vi "RankControls.vi"(6 "error in":errorcluster, 9 "VI Interpreter in":refnum<class "VI Interpreter.lvclass">) -> (0 "error out":errorcluster, 3 "VI Interpreter out":refnum<class "VI Interpreter.lvclass">, 4 "Rank":cluster{"nodes":i32[]}[](array[cluster]))   [LabVIEW 2014, in "Raspberry Pi Compatible Compiler for LabVIEW.lvlib" / "VI Interpreter.lvclass"]
uses:
  VI Interpreter.lvclass
  VI Interpreter.lvclass/VI Interpreter.ctl
  <vilib>/Utility/traverseref.llb/TRef TravTarget.ctl
  VI_AST/VI_AST.lvclass
  VI_AST/VI_AST.lvclass/VI_AST.ctl
  <vilib>/Utility/traverseref.llb/VI Scripting - Traverse.lvlib
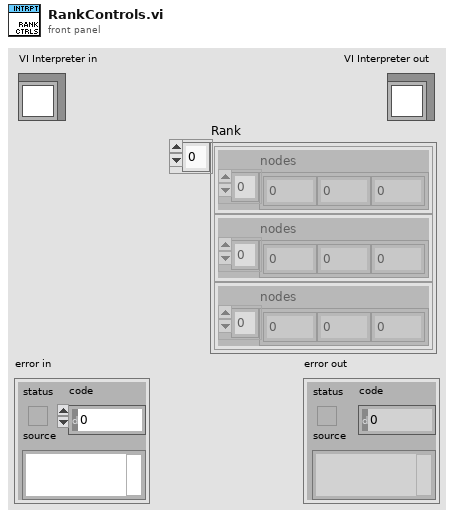
[diagram p1: front panel]
types:
  T1 = typedef "TRef TravTarget.ctl" = enum16{"FP", "BD", "Other"}
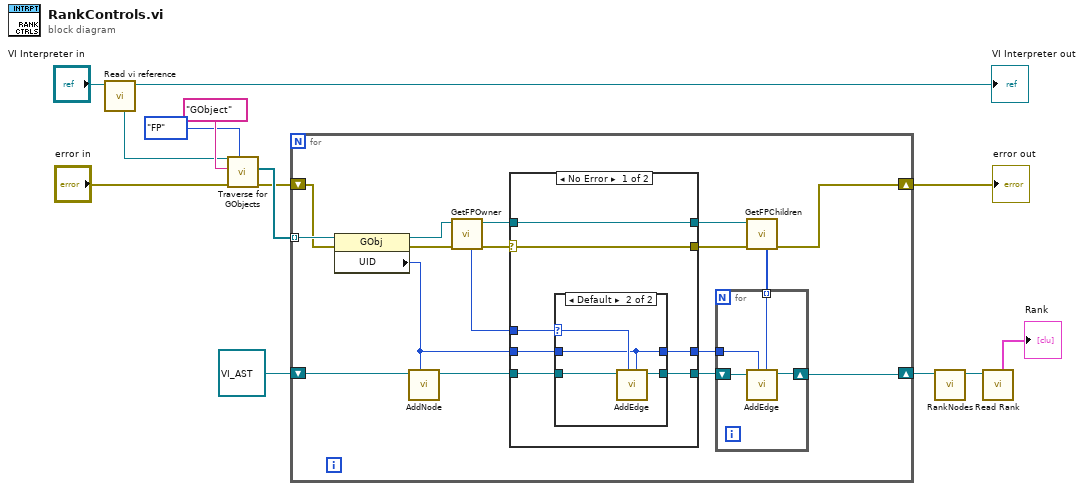
[diagram p0: block diagram]
diagram:
  n1 = call "Read vi reference.vi"("VI Interpreter in"="VI Interpreter in") -> ("VI Interpreter out"=→"VI Interpreter out":refnum<class "VI Interpreter.lvclass">, "vi reference"=w9:refnum<vi>)  [unwired: 7 in]
  n2 = call <vilib>:"Traverse for GObjects.vi"("Traverse Target"=TRef_TravTarget."FP", "error in (no error)"="error in", "Class Name"="GObject", "VI Refnum"=w9) -> ("error out"=w3:errorcluster, "References"=w4:refnum<vi>[])  [unwired: 4 in, 2 out]
  n3 = for {
    tunnel: w4 -> [w23] mode=indexing
    shift-right: [w14] -> w7
    shift-left: refnum<class "VI_AST.lvclass"> refnum ("VI_AST in") -> [w30]
    shift-right: [w18] -> w5
    shift-left: w3 -> [w22]
    n4 = property class="GObj"(reference=w23, error in=w22) -> (reference out=w26:refnum<vi>, error out=w27:errorcluster, "UID"=w28:i32)
    n5 = call "AddNode.vi"("UID"=w28, "VI_AST in"=w30) -> ("VI_AST out"=w29:refnum<class "VI_AST.lvclass">)  [unwired: 6 in, 1 out]
    n6 = call "GetFPOwner.vi"("error in"=w27, "GObj Refnum"=w26) -> ("error out"=w25:errorcluster, "GObj Refnum out"=w20:refnum<vi>, "owner UID"=w24:i32)  [unwired: 5 in]
    n7 = case shown="No Error" w25 {
      selector: w25 -> [w38 _]
      tunnel: [w41 w50] -> w17
      tunnel: w29 -> [w40 w50]
      tunnel: w28 -> [w39 w48]
      tunnel: w24 -> [w37 _]
      tunnel: [w38 _] -> w21
      tunnel: w20 -> [w36 w49]
      tunnel: [w36 w49] -> w19
      tunnel: [w35 w48] -> w15
      frame No Error {
        n8 = case shown="Default" w37 {
          selector: w37 -> [_ w45]
          tunnel: [w43 w47] -> w41
          tunnel: w40 -> [w43 w46]
          tunnel: w39 -> [w42 w44]
          tunnel: [w42 w44] -> w35
          frame 0 {
          }
          frame Default {
            n9 = call "AddEdge.vi"("sink"=w44, "source"=w45, "VI_AST in"=w46) -> ("VI_AST out"=w47:refnum<class "VI_AST.lvclass">)  [unwired: 6 in]
          }
        }
      }
      frame Error {
      }
    }
    n10 = call "GetFPChildren.vi"("error in"=w21, "GObj Refnum"=w19) -> ("error out"=w18:errorcluster, "FP children"=w16:i32[])  [unwired: 5 in, 1 out]
    n11 = for {
      shift-right: [w31] -> w14
      shift-left: w17 -> [w34]
      tunnel: w16 -> [w33] mode=indexing
      tunnel: w15 -> [w32]
      n12 = call "AddEdge.vi"("sink"=w33, "source"=w32, "VI_AST in"=w34) -> ("VI_AST out"=w31:refnum<class "VI_AST.lvclass">)  [unwired: 6 in]
    }
  }
  "error out" <- w5
  n13 = call "RankNodes.vi"("VI_AST in"=w7) -> ("VI_AST out"=w2:refnum<class "VI_AST.lvclass">)  [unwired: 8 in]
  n14 = call "Read Rank.vi"("VI_AST in"=w2) -> ("Rank"=→"Rank":cluster{"nodes":i32[]}[])  [unwired: 7 in, 1 out]
